vi "VISA_WRITE-READ.vi"(4 "WRITE":bool=TRUE, 6 "READ":bool, 7 "Timeout":u32=3000, 8 "error in":errorcluster {"code" format="%.0x"}, 9 "Rcmd":string="RAD:STAN?\n", 10 "Wcmd":string="NONE", 11 "Session In":refnum<visa-resource-name>="TCPIP0::K-N90X0A-00005.local::inst0::INSTR") -> (0 "error out":errorcluster {"code" format="%.0x"}, 3 "Session Out":refnum<visa-resource-name>, 5 "Out":string)   [LabVIEW 2018]
doc: "VISA READ/WRITE Vi"
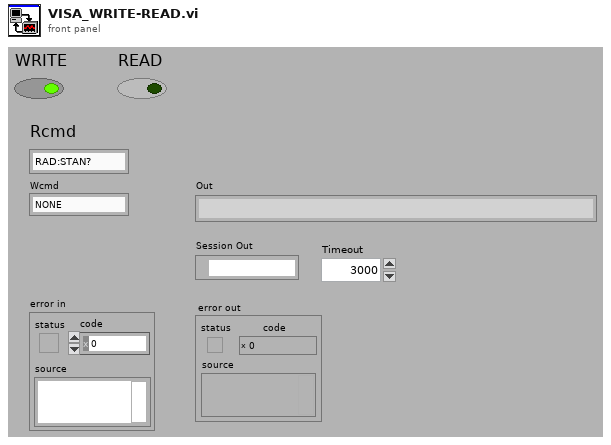
[diagram p1: front panel]
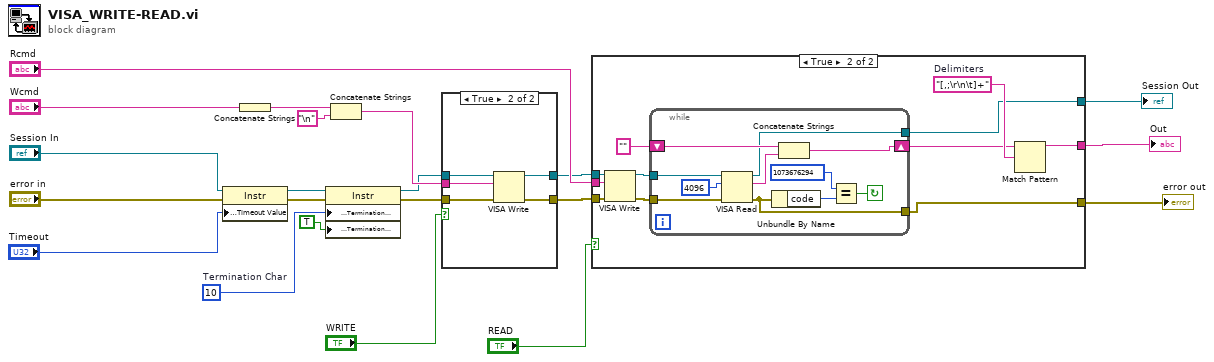
[diagram p0: block diagram]
diagram:
  w16 = u8 10  # Termination Char
  n1 = property class="Instr"(reference="Session In", error in="error in", "General Settings:Timeout Value"="Timeout") -> (reference out=w15:refnum<visa-resource-name>, error out=w18:errorcluster)
  n2 = Concatenate Strings("Wcmd") -> (w10:string)
  n3 = property class="Instr"(reference=w15, error in=w18, "Message Based Settings:Termination Character"=w16, "Message Based Settings:Termination Character Enable"=TRUE ("enable")) -> (reference out=w6:refnum<visa-resource-name>, error out=w17:errorcluster)
  n4 = Concatenate Strings(w10, "\n" ("StaticText")) -> (w11:string)
  n5 = case shown="True" "WRITE" {
    tunnel: w17 -> [w22 w28]
    tunnel: [w22 w27] -> w12
    tunnel: w11 -> [_ w26]
    tunnel: w6 -> [w23 w25]
    tunnel: [w23 w24] -> w5
    frame False {
    }
    frame True {
      n6 = VISA Write(VISA resource name=w25, write buffer=w26, error in (no error)=w28) -> (VISA resource name out=w24:refnum<visa-resource-name>, error out=w27:errorcluster)  [unwired: 1 out]
    }
  }
  n7 = case shown="True" "READ" {
    tunnel: w12 -> [w29 w42]
    tunnel: "Rcmd" -> [w30 w38]
    tunnel: [w30 w37] -> w7
    tunnel: w5 -> [w31 w34]
    tunnel: [w31 w33] -> w4
    tunnel: [w29 w32] -> w3
    frame False {
    }
    frame True {
      w36 = "[,;\r\n\t]+"  # Delimiters
      n8 = VISA Write(VISA resource name=w34, write buffer=w38, error in (no error)=w42) -> (VISA resource name out=w41:refnum<visa-resource-name>, error out=w40:errorcluster)  [unwired: 1 out]
      n9 = while {
        tunnel: w41 -> [w50]
        shift-right: [w44] -> w35
        shift-left: "" -> [w49]
        tunnel: w40 -> [w47]
        tunnel: [w46] -> w32
        tunnel: [w43] -> w33
        stop <- w45 continue-if-true
        n10 = VISA Read(VISA resource name=w50, byte count=u32 4096 ("byte count (0)"), error in (no error)=w47) -> (VISA resource name out=w43:refnum<visa-resource-name>, read buffer=w48:string, error out=w46:errorcluster)  [unwired: 1 out]
        n11 = Unbundle By Name(w46) -> ("code"=w52:i32)
        n12 = Concatenate Strings(w49, w48) -> (w44:string)
        n13 = Equal?(x=1073676294, y=w52) -> (x = y?=w45:bool)
      }
      n14 = Match Pattern(string=w35, regular expression=w36) -> (before substring=w37:string)  [unwired: 4 out]
    }
  }
  "Out" <- w7
  "Session Out" <- w4
  "error out" <- w3
